vi "XYtoRPHI.vi"(1 "X-Y":dbl[](array[numeric])) -> (0 "r-phi":dbl[](array[numeric]))   [LabVIEW 2016]
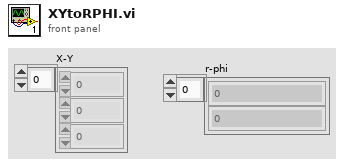
[diagram p1: front panel]
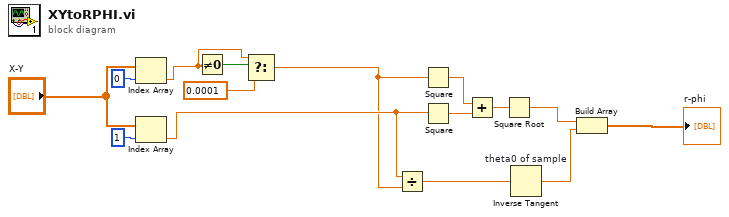
[diagram p0: block diagram]
diagram:
  n1 = Index Array(array="X-Y", index=0) -> (element=w3:dbl)
  n2 = Index Array(array="X-Y", index=1) -> (element=w8:dbl)
  n3 = Not Equal To 0?(x=w3) -> (x != 0?=w4:bool)
  n4 = Select(t=w3, s=w4, f=0.0001) -> (s? t:f=w1:dbl)
  n5 = Divide(x=w8, y=w1) -> (x/y=w9:dbl)
  n6 = Square(x=w1) -> (x^2=w12:dbl)
  n7 = Square(x=w8) -> (x^2=w13:dbl)
  n8 = Add(x=w12, y=w13) -> (x+y=w11:dbl)
  n9 = Square Root(x=w11) -> (sqrt(x)=w7:dbl)
  n10 = Inverse Tangent "theta0 of sample"(1:w9) -> (0:w6:dbl)
  n11 = Build Array(w7, w6) -> (→"r-phi":dbl[])
